vi "ReverseThreshold_Automatic.vi"(4 "Error IN Toolkit":i32, 5 "Error IN LabVIEW":errorcluster, 6 "min":u8, 8 "max":u8) -> (18 "Error OUT Toolkit":i32, 19 "Error OUT LabVIEW":errorcluster)   [LabVIEW 2018]
doc: "Binarize an image (previously converted to 1D Array U8) to separate the internal elements, based on a thresholding, converting the pixels from inside and 0s from outside the threshold to 1s. It receives a minimum and a maximum for the range.\n\nFor correct operation it should receive an error that comes from a VI of some processing algorithm or that contains a copy data of CPU-GPU."
uses:
  dll/LibreriaAutis_3.dll
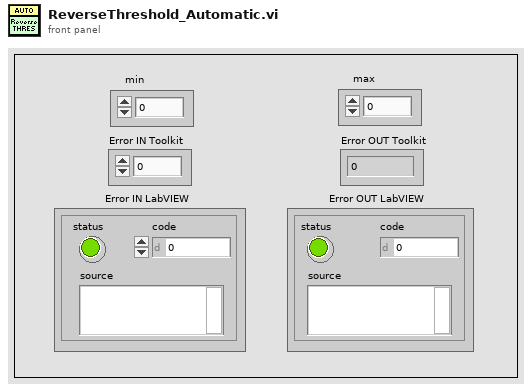
[diagram p1: front panel]
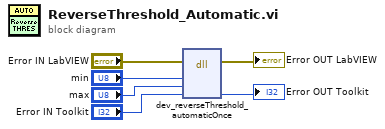
[diagram p0: block diagram]
diagram:
  n1 = dll-call lib="C:/Users/AUTIS/Desktop/LibreriaAUTIS/LabVIEW/dll/LibreriaAutis_3.dll" fn="dev_reverseThreshold_automaticOnce"(error in="Error IN LabVIEW", "min"="min", "max"="max", "error"="Error IN Toolkit") -> (error out=→"Error OUT LabVIEW":errorcluster, "error"=→"Error OUT Toolkit":i32)  [unwired: 5 in, 1 out]
